vi "Set LV TCP-IP Server Port.vi"(8 "error in (no error)":errorcluster) -> (0 "error out":errorcluster)   [LabVIEW 2016]
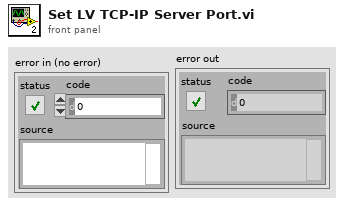
[diagram p1: front panel]
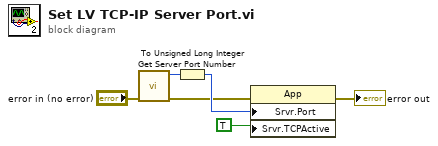
[diagram p0: block diagram]
diagram:
  n1 = call "Get Server Port Number.vi"("error in (no error)"="error in (no error)") -> ("error out"=w3:errorcluster, "Server Port"=w6:u16)  [unwired: 8 in, 1 out]
  n2 = To Unsigned Long Integer(number=w6) -> (unsigned 32bit integer=w5:u32)
  n3 = property class="App"(error in=w3, "Srvr.Port"=w5, "Srvr.TCPActive"=TRUE ("Server:TCP Listener Active")) -> (error out=→"error out":errorcluster)  [unwired: 1 in, 1 out]
